vi "DKL_Labview_interface.vi"() -> ()   [LabVIEW 2018]
uses:
  <vilib>/Utility/file.llb/Write Delimited Spreadsheet (string).vi
panel:
  in  "Linear Subtract (F = Raw)":bool=TRUE
  out "Frame x,y (nm)":dbl[](array[numeric])
  out "Subimage patches":dbl
  in  "Window size":i16
  in  "Coordinate step":i16
  in  "Iterations":i32
  in  "stop":bool
  out "Current iteration":i32
  out "Scalar value":dbl
  out "compilation_file":string
  out "Waveform Graph":dbl[](graph)
  in  "Experiment Name":string
  in  "Data Direction:\n Fwd/Bwd (T=Fwd)":bool=TRUE
  in  "Scan Direction: (T=down-top) 3":bool=TRUE
  out "error out":errorcluster
  out "Application ref out":refnum<vi>
  out "Go to point (nm)":dbl[](array[numeric])
  in  "Spectroscopy Parameter 2":cluster{"Start":dbl, "Stop":dbl, "# Points":i32}={"Start"=-2.0, "Stop"=2.0, "# Points"=256} {"# Points" min=2; "Stop" format="%1_3p"; "Start" format="%1_3p"}
  in  "Error in (no error)":errorcluster
  # "Spectroscopy"
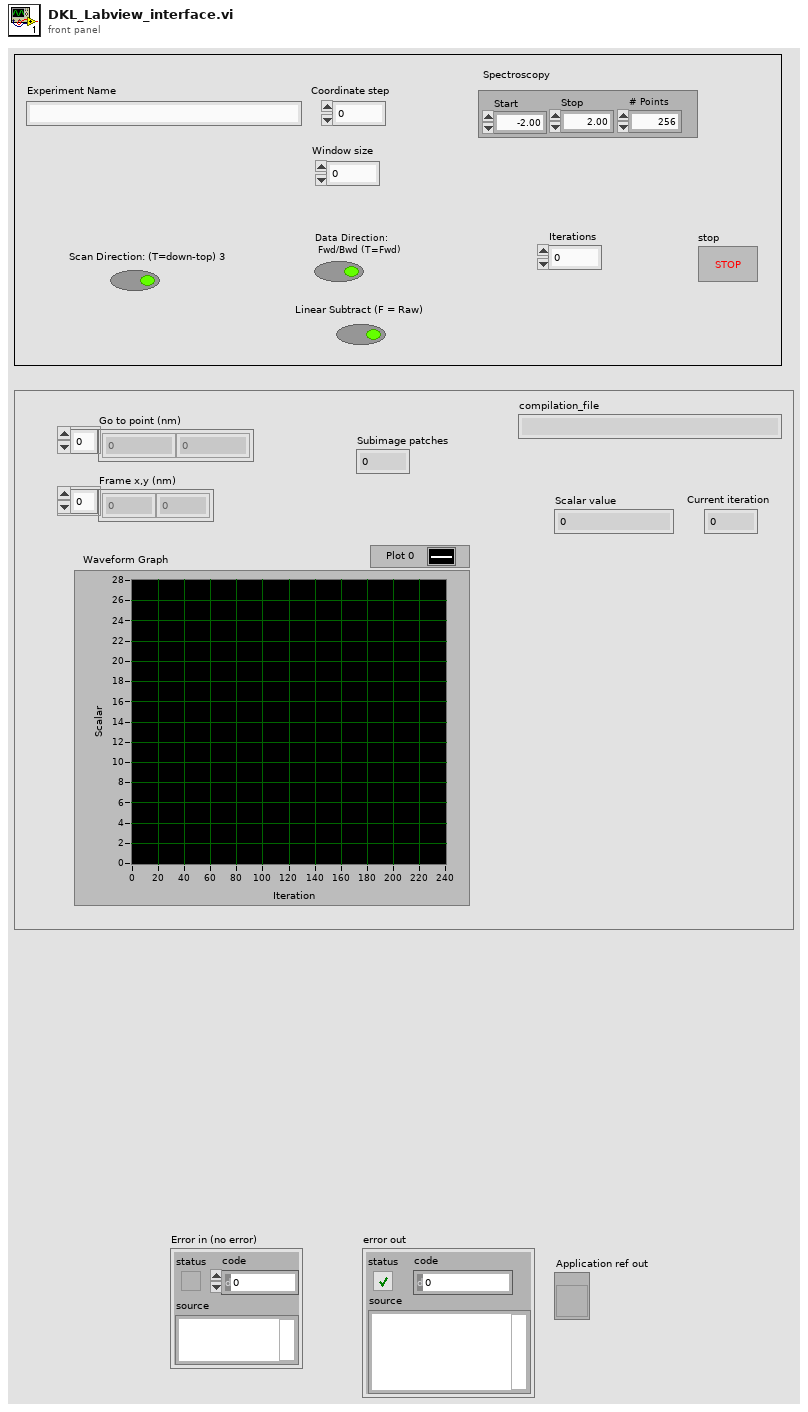
[diagram p1: front panel]
types:
  T1 = enum16{"open", "replace", "create", "open or create", "replace or create", "replace or create with confirmation"}
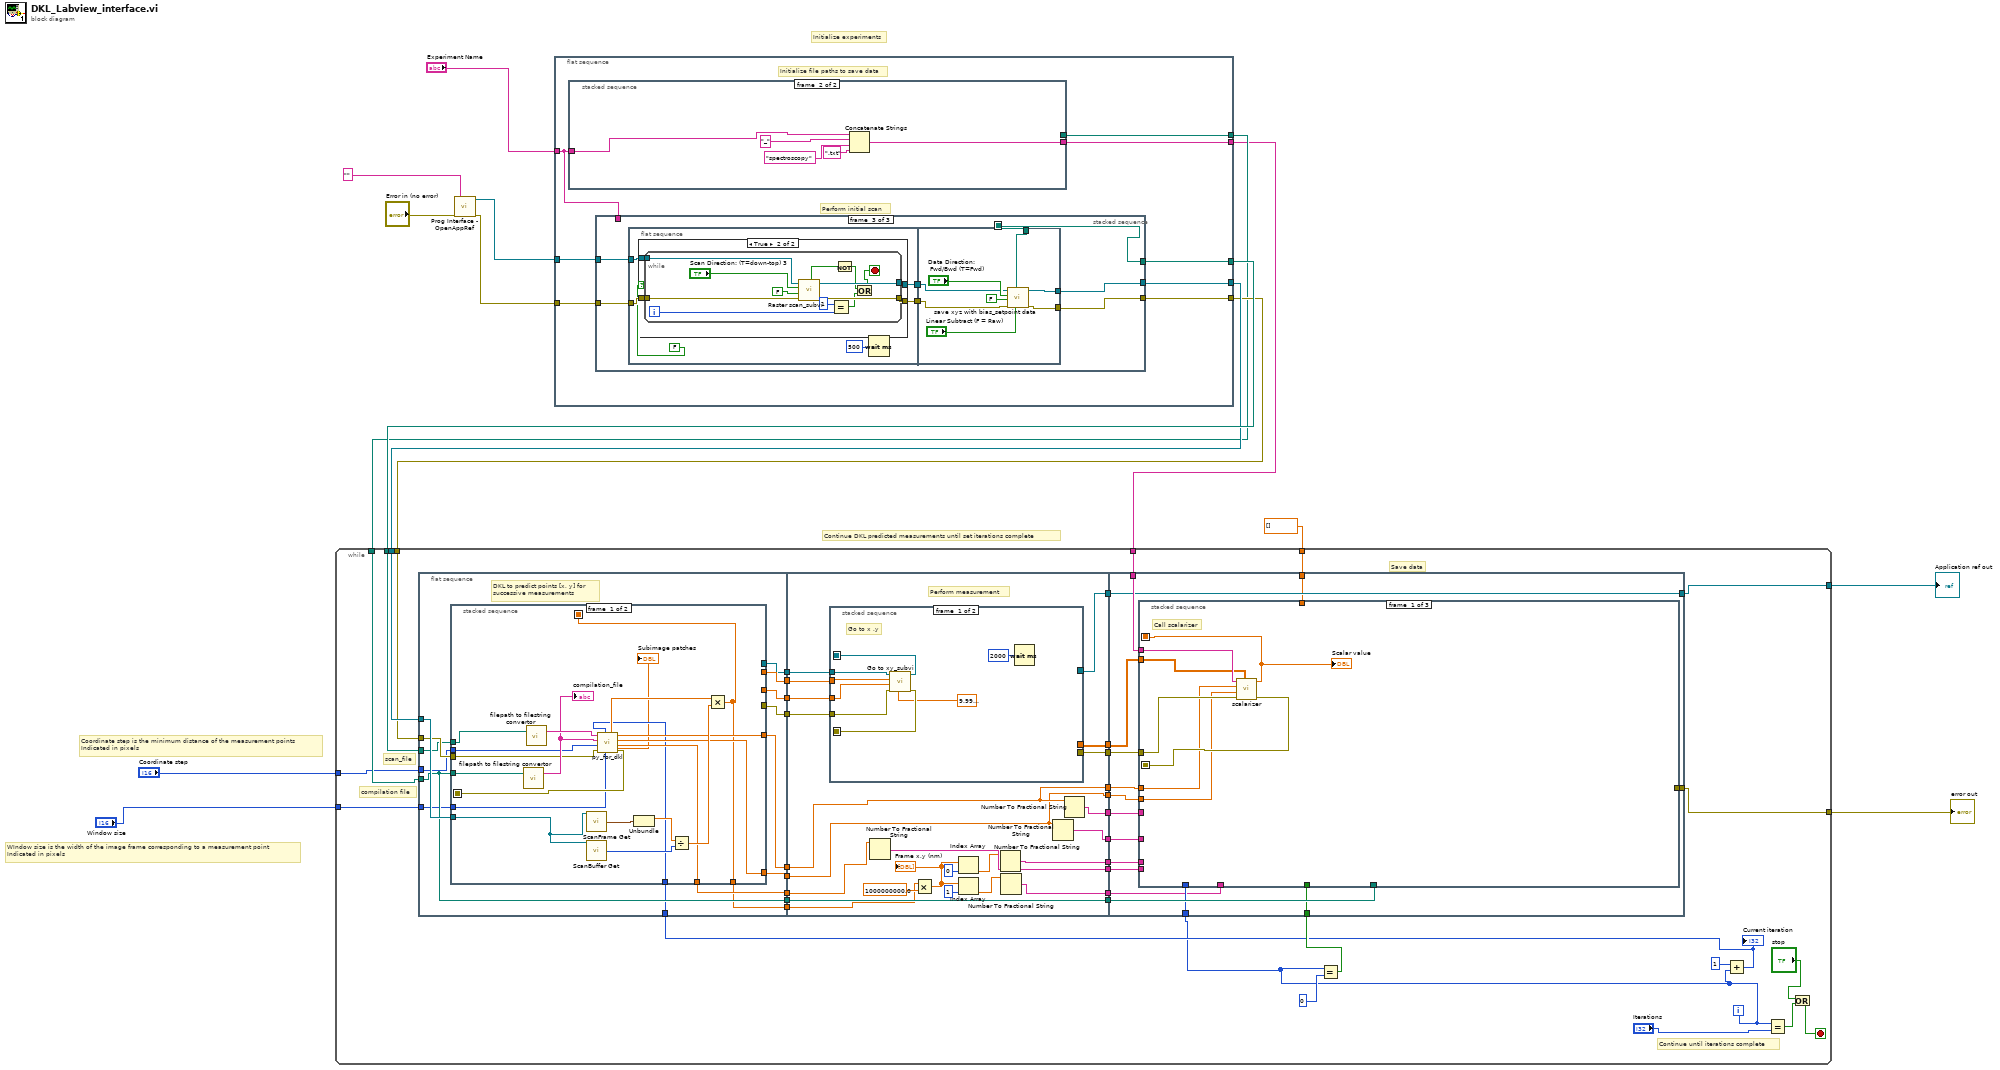
[diagram p0: block diagram]
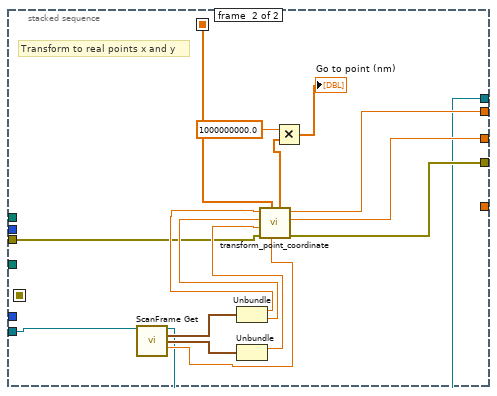
[diagram p2: hidden frame]
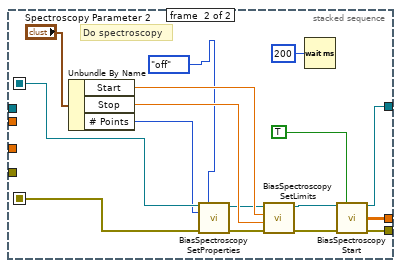
[diagram p3: hidden frame]
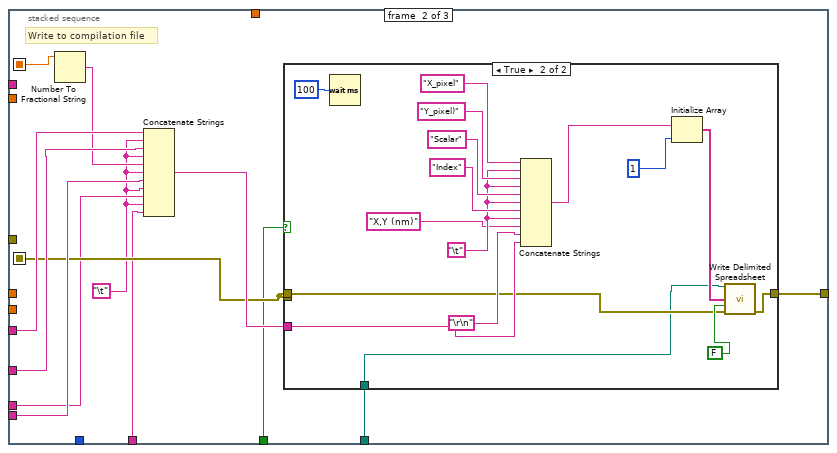
[diagram p4: hidden frame]
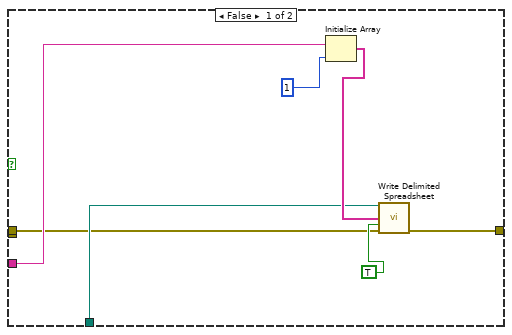
[diagram p5: hidden frame]
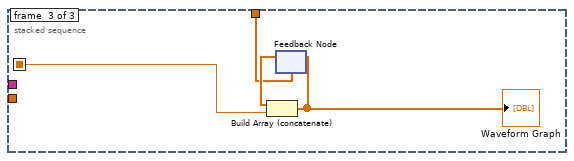
[diagram p6: hidden frame]
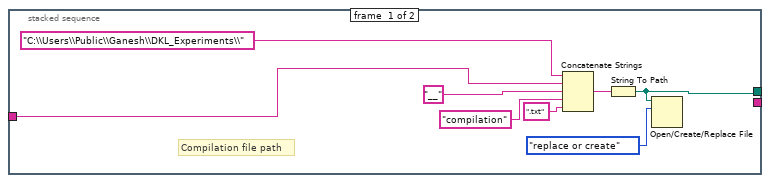
[diagram p7: hidden frame]
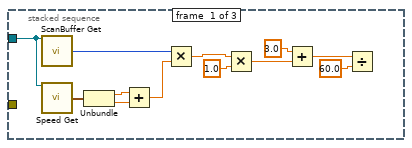
[diagram p8: hidden frame]
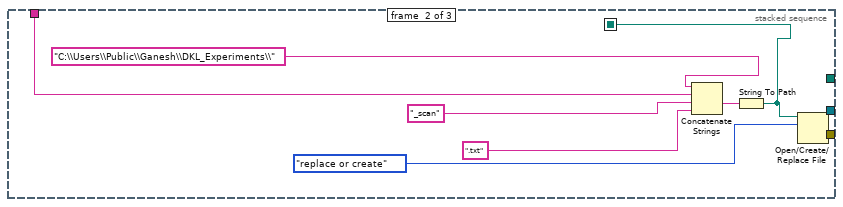
[diagram p9: hidden frame]
diagram:
  # "Continue DKL predicted measurements until set iterations complete"
  # "Initialize experiments"
  # "WIndow size is the width of the image frame corresponding to a measurement point\nIndicated in pixels"
  # "Coordinate step is the minimum distance of the measurement points\nIndicated in pixels"
  n1 = while {
    tunnel: w11 -> [w54]
    tunnel: w10 -> [w53]
    tunnel: w9 -> [w52]
    tunnel: w8 -> [w51]
    tunnel: w7 -> [w45]
    tunnel: [w31] -> w6
    tunnel: [w30] -> w5
    tunnel: "Coordinate step" -> [w22]
    tunnel: "Window size" -> [w21]
    tunnel: dbl[] [] -> [w20]
    i -> [w16]
    stop <- w27 stop-if-true
    # "Continue until iterations complete"
    # "Save data"
    # "scan_file"
    # "compilation file"
    n2 = flat-sequence {
      tunnel: w51 -> [w62]
      tunnel: w54 -> [w67]
      tunnel: w53 -> [w69]
      tunnel: w52 -> [w68]
      tunnel: [w66] -> w50
      tunnel: [w65] -> w49
      tunnel: [w64] -> w48
      tunnel: [w63] -> w47
      tunnel: [w62] -> w42
      tunnel: [w61] -> w41
      tunnel: [w60] -> w40
      tunnel: [w59] -> w39
      tunnel: [w58] -> w35
      tunnel: w22 -> [w57]
      tunnel: w17 -> [w56]
      tunnel: w21 -> [w55]
      tunnel: w50 -> [w128]
      tunnel: w49 -> [w127]
      tunnel: w48 -> [w126]
      tunnel: w47 -> [w125]
      tunnel: [w124] -> w46
      tunnel: [w123] -> w44
      tunnel: [w122] -> w43
      tunnel: w42 -> [w122]
      tunnel: w41 -> [w121]
      tunnel: w40 -> [w107]
      tunnel: w39 -> [w106]
      tunnel: [w109] -> w38
      tunnel: [w108] -> w37
      tunnel: [w120] -> w36
      tunnel: w35 -> [w118]
      tunnel: [w117] -> w34
      tunnel: [w111] -> w25
      tunnel: [w110] -> w24
      tunnel: [w107] -> w19
      tunnel: [w106] -> w18
      tunnel: w46 -> [w168]
      tunnel: w45 -> [w167]
      tunnel: w44 -> [w166]
      tunnel: w43 -> [w162]
      tunnel: w38 -> [w165]
      tunnel: w37 -> [w164]
      tunnel: w36 -> [w163]
      tunnel: w34 -> [w160]
      tunnel: w32 -> [w161]
      tunnel: [w160] -> w31
      tunnel: [w159] -> w30
      tunnel: w16 -> [w158]
      tunnel: w25 -> [w157]
      tunnel: w24 -> [w156]
      tunnel: w20 -> [w155]
      tunnel: w19 -> [w154]
      tunnel: w18 -> [w153]
      frame #0 {
        # "DKL to predict points [x, y] for \nsuccessive measurements"
        n3 = stacked-sequence {
          seq-local: [w74 _] -> [_ w104]
          seq-local: [w79 _] -> [_ _]
          tunnel: w69 -> [w78 w105]
          tunnel: w68 -> [w80 w97]
          tunnel: w67 -> [w89 _]
          tunnel: w62 -> [w88 _]
          tunnel: [_ w96] -> w66
          tunnel: [_ w95] -> w65
          tunnel: [_ w94] -> w64
          tunnel: [_ w93] -> w63
          tunnel: [w77 _] -> w61
          tunnel: [w76 _] -> w60
          tunnel: [w75 _] -> w59
          tunnel: [w74 _] -> w58
          tunnel: w57 -> [w73 _]
          tunnel: w56 -> [w72 _]
          tunnel: w55 -> [w71 _]
          frame #0 {
            n4 = call "filepath to filestring convertor.vi"("path"=w88) -> ("element"=w86:string)  [unwired: 2 in]
            "compilation_file" <- w86
            n5 = call "filepath to filestring convertor.vi"("path"=w89) -> ("element"=w87:string)  [unwired: 2 in]
            n6 = call "ScanFrame Get.vi"("Application ref in"=w78) -> ("Size (m)"=w85:cluster{"Width":sgl, "Height":sgl})  [unwired: 10 in, 4 out]
            n7 = call "ScanBuffer Get.vi"("Application ref in"=w78) -> ("Pixels/line"=w83:i32)  [unwired: 10 in, 4 out]
            n8 = call "py_for_dkl.vi"("Window size"=w71, "Iteration_no"=w72, "error in (no error)"=w80, "Coordinate step"=w73, "Compilation_file_name"=w86, "Scan_file_name"=w87) -> ("error out"=w79:errorcluster, "index"=w77:dbl, "pixel_y"=w75:dbl, "pixel_x"=w76:dbl, "Subimage patches"=→"Subimage patches":dbl, "Pixels (x,y)"=w81:dbl[])
            n9 = Unbundle(w85) -> ("Width"=w84:sgl)  [unwired: 1 out]
            n10 = Divide(x=w84, y=w83) -> (x/y=w82:sgl)
            n11 = Multiply(x=w81, y=w82) -> (x*y=w74:dbl[])
          }
          frame #1 {
            # "Transform to real points x and y"
            n12 = call "ScanFrame Get.vi"("Application ref in"=w105) -> ("Application ref out"=w93:refnum<vi>, "Center coordinates (m)"=w103:cluster{"Xc":sgl, "Yc":sgl}, "Size (m)"=w102:cluster{"Width":sgl, "Height":sgl}, "Angle (deg)"=w98:sgl)  [unwired: 10 in, 1 out]
            n13 = Unbundle(w103) -> ("Xc"=w101:sgl, "Yc"=w100:sgl)
            n14 = Unbundle(w102) -> ("Width"=w99:sgl)  [unwired: 1 out]
            n15 = call "transform_point_coordinate.vi"("Angle (deg)"=w98, "i/p Point Array (x,y)"=w104, "error in (no error)"=w97, "Frame_length"=w99, "Yc"=w100, "Xc"=w101) -> ("error out"=w94:errorcluster, "transform_y"=w95:dbl, "transform_x"=w96:dbl, "transform point (x,y)"=w91:dbl[])  [unwired: 2 in]
            n16 = Multiply(x=1000000000.0, y=w91) -> (x*y=→"Go to point (nm)":dbl[])
          }
        }
      }
      frame #1 {
        # "Perform measurement"
        n17 = stacked-sequence {
          seq-local: [w131 _] -> [_ w146]
          seq-local: [w132 _] -> [_ w145]
          tunnel: w128 -> [w134 _]
          tunnel: w127 -> [w133 _]
          tunnel: w126 -> [w136 _]
          tunnel: w125 -> [w135 _]
          tunnel: [_ w141] -> w124
          tunnel: [_ w140] -> w123
          tunnel: [_ w139] -> w117
          frame #0 {
            # "Go to x ,y"
            n18 = call "Go to xy_subvi.vi"("Speed (m/s)"=sgl 1e-09, "error in (no error)"=w136, "Y (m)"=w133, "X (m)"=w134, "Application ref in"=w135) -> ("error out"=w132:errorcluster, "Application ref out"=w131:refnum<vi>)  [unwired: 5 in]
            n19 = Wait (ms)(milliseconds to wait=u32 2000) -> ()  [unwired: 1 out]
          }
          frame #1 {
            # "Do spectroscopy"
            n20 = Unbundle By Name("Spectroscopy Parameter 2") -> ("Start"=w149:dbl, "Stop"=w148:dbl, "# Points"=w142:i32)
            n21 = call "BiasSpectroscopy SetProperties.vi"("Application ref in"=w146, "Backward sweep (no change)"=enum16{"no change", "on", "off"}."off", "Number of points (0=no change)"=w142, "Error in (no error)"=w145) -> ("Application ref out"=w144:refnum<vi>, "Error out"=w143:errorcluster)  [unwired: 10 in]
            n22 = call "BiasSpectroscopy SetLimits.vi"("Error in (no error)"=w143, "End value (V)"=w148, "Start value (V)"=w149, "Application ref in"=w144) -> ("Error out"=w152:errorcluster, "Application ref out"=w151:refnum<vi>)  [unwired: 4 in]
            n23 = Wait (ms)(milliseconds to wait=u32 200) -> ()  [unwired: 1 out]
            n24 = call "BiasSpectroscopy Start.vi"("Application ref in"=w151, "Get data (F)"=TRUE, "Error in (no error)"=w152) -> ("Application ref out"=w139:refnum<vi>, "Data"=w141:sgl[][], "Error out"=w140:errorcluster)  [unwired: 8 in, 2 out]
          }
        }
        n25 = Number To Fractional String(number=w121) -> (F-format string=w120:string)  [unwired: 3 in]
        n26 = Multiply(x=w118, y=1000000000.0) -> (x*y=w116:dbl[])
        "Frame x,y (nm)" <- w116
        n27 = Index Array(array=w116, index=0) -> (element=w113:dbl)
        n28 = Index Array(array=w116, index=1) -> (element=w112:dbl)
        n29 = Number To Fractional String(number=w113) -> (F-format string=w110:string)  [unwired: 3 in]
        n30 = Number To Fractional String(number=w112) -> (F-format string=w111:string)  [unwired: 3 in]
        n31 = Number To Fractional String(number=w106) -> (F-format string=w108:string)  [unwired: 3 in]
        n32 = Number To Fractional String(number=w107) -> (F-format string=w109:string)  [unwired: 3 in]
      }
      frame #2 {
        n33 = stacked-sequence {
          seq-local: [w173 _ _] -> [_ w181 _]
          seq-local: [w172 _ _] -> [_ w188 w215]
          tunnel: w168 -> [w171 _ _]
          tunnel: w167 -> [w175 _ _]
          tunnel: w166 -> [w174 _ _]
          tunnel: w165 -> [_ w187 _]
          tunnel: w164 -> [_ w186 _]
          tunnel: w163 -> [_ w184 _]
          tunnel: w162 -> [_ w182 _]
          tunnel: w161 -> [_ w180 _]
          tunnel: [_ w179 _] -> w159
          tunnel: w158 -> [_ _ _]
          tunnel: w157 -> [_ w178 _]
          tunnel: w156 -> [_ w177 _]
          tunnel: w155 -> [_ _ w212]
          tunnel: w154 -> [w170 _ _]
          tunnel: w153 -> [w169 _ _]
          frame #0 {
            # "Call scalarizer"
            n34 = call "scalarizer.vi"("Array"=w171, "error in (no error)"=w174, "pixel_y"=w169, "pixel_x"=w170, "Spectroscopy_file"=w175) -> ("error out"=w173:errorcluster, "return value"=w172:dbl)  [unwired: 5 in]
            "Scalar value" <- w172
          }
          frame #1 {
            w176 = "\t"
            # "Write to compilation file"
            n35 = Number To Fractional String(number=w188) -> (F-format string=w185:string)  [unwired: 3 in]
            n36 = Concatenate Strings(w187, w176, w186, w176, w185, w176, w184, w176, w177, w176, w178) -> (w183:string)
            n37 = case shown="True" w180 {
              tunnel: w183 -> [w193 w199]
              tunnel: w182 -> [w191 w197]
              tunnel: w181 -> [_ _]
              tunnel: w181 -> [w190 w198]
              tunnel: [w189 w196] -> w179
              frame False {
                n38 = Initialize Array(w193, 1 ("dimension size")) -> (w192:string[])
                n39 = call-poly <vilib>:"Write Delimited Spreadsheet.vi"("file path (dialog if empty)"=w191, "1D data"=w192, "append to file? (new file:F)"=TRUE, "error in (no error)"=w190) -> ("error out"=w189:errorcluster)  [unwired: 10 in, 1 out]
              }
              frame True {
                w202 = "\t"
                n40 = Wait (ms)(milliseconds to wait=u32 100) -> ()  [unwired: 1 out]
                n41 = Concatenate Strings("X_pixel" ("string"), w202, "Y_pixel)" ("string"), w202, "Scalar" ("string"), w202, "Index" ("string"), w202, "X,Y (nm)" ("string"), "\r\n", w199) -> (w207:string)
                n42 = Initialize Array(w207, 1 ("dimension size")) -> (w206:string[])
                n43 = call-poly <vilib>:"Write Delimited Spreadsheet.vi"("file path (dialog if empty)"=w197, "1D data"=w206, "append to file? (new file:F)"=FALSE, "error in (no error)"=w198) -> ("error out"=w196:errorcluster)  [unwired: 10 in, 1 out]
              }
            }
          }
          frame #2 {
            n44 = feedback #1(w212) -> (w214:dbl[])
            n45 = Build Array (concatenate)(w214, w215) -> (w213:dbl[])
            "Waveform Graph" <- w213
            n46 = feedback-in #1(w213) -> ()
          }
        }
      }
    }
    n47 = Equal?(x=w16, y=0) -> (x = y?=w32:bool)
    n48 = Add(x=1, y=w16) -> (x+y=w17:i32)
    "Current iteration" <- w17
    n49 = Equal?(x=w16, y="Iterations") -> (x = y?=w29:bool)
    n50 = Or(x="stop", y=w29) -> (x .or. y?=w27:bool)
  }
  "Application ref out" <- w6
  "error out" <- w5
  n51 = call "Prog Interface - OpenAppRef.vi"("Error in (no error)"="Error in (no error)", "Machine name (local machine IP)"="") -> ("Error out"=w13:errorcluster, "Application reference"=w14:refnum<vi>)  [unwired: 4 in]
  n52 = flat-sequence {
    tunnel: w14 -> [w223]
    tunnel: w13 -> [w220]
    tunnel: "Experiment Name" -> [w219]
    tunnel: [w222] -> w10
    tunnel: [w221] -> w9
    tunnel: [w218] -> w8
    tunnel: [w217] -> w11
    tunnel: [w216] -> w7
    frame #0 {
      # "Perform initial scan"
      # "Initialize file paths to save data"
      n53 = stacked-sequence {
        tunnel: [w225 _] -> w218
        tunnel: w219 -> [w224 w233]
        tunnel: [_ w232] -> w216
        frame #0 {
          # "Compilation file path"
          n54 = Concatenate Strings("C:\\Users\\Public\\Ganesh\\DKL_Experiments\\", w224, "__" ("string"), "compilation" ("string"), ".txt" ("string")) -> (w229:string)
          n55 = String To Path(string=w229) -> (path=w225:path)
          n56 = Open/Create/Replace File(file path (use dialog)=w225, operation (0:open)=T1."replace or create") -> ()  [unwired: 4 in, 3 out]
        }
        frame #1 {
          n57 = Concatenate Strings(w233, "_" ("string"), "spectroscopy" ("string"), ".txt" ("string")) -> (w232:string)
        }
      }
      n58 = stacked-sequence {
        seq-local: [_ w250 _] -> [_ _ w258]
        tunnel: w223 -> [w243 _ w262]
        tunnel: [_ _ w256] -> w222
        tunnel: [_ _ w257] -> w221
        tunnel: w220 -> [_ _ w261]
        tunnel: w219 -> [_ w251 _]
        tunnel: [_ _ w258] -> w217
        frame #0 {
          n59 = call "ScanBuffer Get.vi"("Application ref in"=w243) -> ("Pixels/line"=w247:i32)  [unwired: 10 in, 4 out]
          n60 = call "Speed Get.vi"("Application ref in"=w243) -> ("Time/line (s)"=w248:cluster{"Forward":sgl, "Backward":sgl})  [unwired: 9 in, 5 out]
          n61 = Unbundle(w248) -> ("Forward"=w246:sgl, "Backward"=w245:sgl)
          n62 = Add(x=w246, y=w245) -> (x+y=w244:sgl)
          n63 = Multiply(x=w247, y=w244) -> (x*y=w242:sgl)
          n64 = Multiply(x=w242, y=sgl 1.0) -> (x*y=w240:sgl)
          n65 = Add(x=3.0, y=w240) -> (x+y=w238:dbl)
          n66 = Divide(x=w238, y=60.0) -> ()  [unwired: 1 out]
        }
        frame #1 {
          n67 = Concatenate Strings("C:\\Users\\Public\\Ganesh\\DKL_Experiments\\", w251, "_scan" ("string"), ".txt" ("string")) -> (w253:string)
          n68 = String To Path(string=w253) -> (path=w250:path)
          n69 = Open/Create/Replace File(file path (use dialog)=w250, operation (0:open)=T1."replace or create") -> ()  [unwired: 4 in, 3 out]
        }
        frame #2 {
          n70 = flat-sequence {
            tunnel: w262 -> [w267]
            tunnel: w261 -> [w266]
            tunnel: [w268] -> w260
            tunnel: [w265] -> w259
            tunnel: w260 -> [w291]
            tunnel: w259 -> [w289]
            tunnel: w258 -> [w292]
            tunnel: [w288] -> w257
            tunnel: [w287] -> w256
            frame #0 {
              n71 = case shown="True" FALSE {
                tunnel: [w270 w274] -> w268
                tunnel: w267 -> [w269 w273]
                tunnel: w266 -> [w270 w272]
                tunnel: [w269 w271] -> w265
                frame False {
                }
                frame True {
                  n72 = while {
                    tunnel: w273 -> [w283]
                    tunnel: w272 -> [w286]
                    tunnel: [w282] -> w271
                    tunnel: [w281] -> w274
                    i -> [w279]
                    stop <- w275 stop-if-true
                    n73 = call "Raster scan_subvi.vi"("error in (no error)"=w286, "Draw Outline"=FALSE, "Direction: (T=down-top)"="Scan Direction: (T=down-top) 3", "Application ref in"=w283) -> ("error out"=w281:errorcluster, "Application ref out"=w282:refnum<vi>, "Scan status"=w284:bool)  [unwired: 1 in, 4 out]
                    n74 = Equal?(x=1, y=w279) -> (x = y?=w277:bool)
                    n75 = Not(x=w284) -> (.not. x?=w276:bool)
                    n76 = Or(x=w276, y=w277) -> (x .or. y?=w275:bool)
                  }
                }
              }
              n77 = Wait (ms)(milliseconds to wait=u32 500) -> ()  [unwired: 1 out]
            }
            frame #1 {
              n78 = call "save xyz with bias_setpoint data.vi"("Linear Subtract (F = Raw)"="Linear Subtract (F = Raw)", "file path (dialog if empty)"=w292, "error in (no error)"=w291, "append to file? (new file:F)"=FALSE, "Direction: Fwd/Bwd (T=Fwd)"="Data Direction:\n Fwd/Bwd (T=Fwd)", "Application ref in"=w289) -> ("error out"=w288:errorcluster, "Application ref out"=w287:refnum<vi>)  [unwired: 4 in]
            }
          }
        }
      }
    }
  }
